vi "Queue Cooms FGV.vi"(8 "error in":errorcluster, 10 "Action":T1, 11 "queue in":refnum<queue>) -> (0 "error out":errorcluster, 3 "queue out":refnum<queue>)   [LabVIEW 2019]
doc: "Este VI es una FGV que provee al módulo acceso a la cola."
uses:
  Private Controls/Queue FGV Action.ctl
  Private Controls/Control HMI Data Cluster.ctl
  Private Controls/Estados.ctl
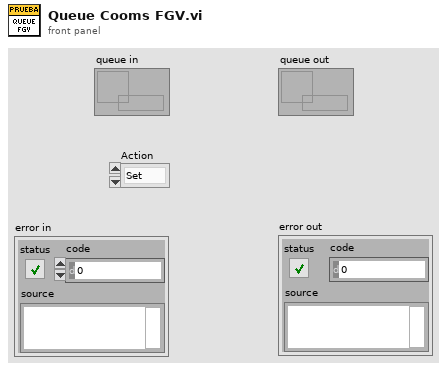
[diagram p1: front panel]
types:
  T1 = typedef "Queue FGV Action.ctl" = enum16{"Set", "Get", "Release"}
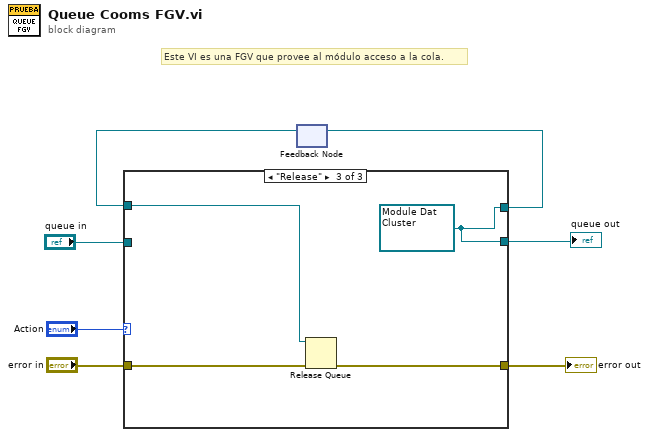
[diagram p0: block diagram]
diagram:
  # "Este VI es una FGV que provee al módulo acceso a la cola."
  n1 = feedback #1() -> (w5:refnum<queue>)  [unwired: 1 in]
  n2 = case shown="\"Release\"" "Action" {
    tunnel: [w8 w11 w13] -> w1
    tunnel: [w8 w11 w13] -> w6
    tunnel: w5 -> [_ w11 w12]
    tunnel: "error in" -> [w9 w10 w15]
    tunnel: [w9 w10 w14] -> w4
    tunnel: "queue in" -> [w8 _ _]
    frame "Set", Default {
    }
    frame "Get" {
    }
    frame "Release" {
      w13 = refnum<queue> refnum ("queue out")
      n3 = Release Queue(queue=w12, error in (no error)=w15) -> (error out=w14:errorcluster)  [unwired: 1 in, 2 out]
    }
  }
  "error out" <- w4
  "queue out" <- w1
  n4 = feedback-in #1(w6) -> ()
